vi "Secure-Release Region_01282025.vi"(6 "Numeric":dbl, 7 "Action":enum16{"Secure", "Release"}(ring), 8 "error in (no error)":errorcluster, 10 "Control In":T1={"I-O.lvclass"=refnum, "Gantry"=refnum, "Dispenser"="COM1"}, 11 "Carrier Tray in":refnum<class "Assembly Tray.lvclass">) -> (0 "error out":errorcluster, 1 "Position":i32, 2 "Control Out":T1={"I-O.lvclass"=refnum, "Gantry"=refnum, "Dispenser"="COM1"}, 3 "Carrier Tray out":refnum<class "Assembly Tray.lvclass">)   [LabVIEW 2021, in "Assembly Tray.lvclass"]
uses:
  Assembly Tray.lvclass
  C:/Users/User/Documents/Jessica_Code/Jessica_code_08062024/Gantry-CMU/UCSB-Gantry-HEP-main/Classes/Workspace/Fixture.lvclass
  Controller/Controllers.ctl
  Controller/I-O/I-O.lvclass
  C:/Program Files (x86)/Aerotech/A3200/LabVIEW/2010/Bin/Aerotech.A3200.dll
  Program Files (x86)/Aerotech/A3200/LabVIEW/2010/Bin/Aerotech.A3200.dll
  Fixture.lvclass/Fixture.ctl
  Assembly Tray.lvclass/Assembly Tray.ctl
  Fixture.lvclass
  Controller/Controller.lvclass
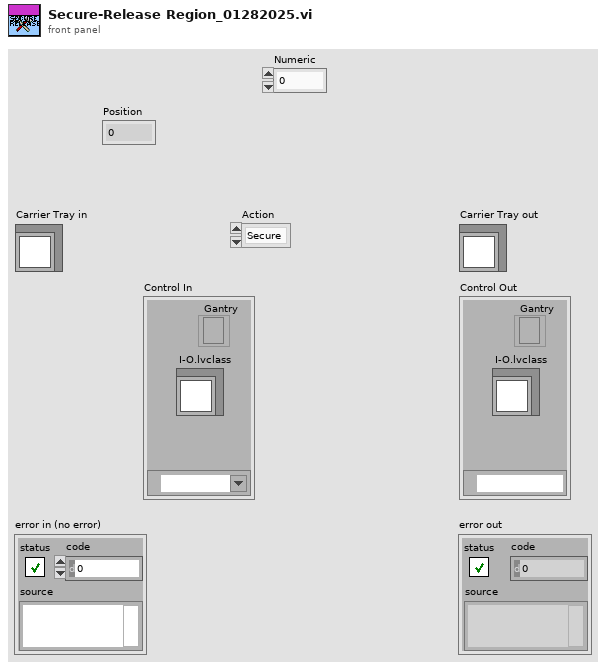
[diagram p1: front panel]
types:
  T1 = typedef "Controller.lvclass/Controllers.ctl" = cluster{"I-O.lvclass":refnum<class "I-O.lvclass">, "Gantry":refnum<k24>, "Dispenser":refnum<visa-resource-name>}
  T2 = typedef "I-O.lvclass/Pin Map.ctl" = cluster{"Region Valves":i32[], "Extra Valves":dbl[][][], "Tool Primary Valve":i32, "Tool Secondary Valve":i32, "Region Sensors":i32[], "Extra Sensors":dbl[][][], "Tool Primary Sensor":dbl, "Tool Secondary Sensor":dbl, "Compression Sensor":dbl, "5V":i32, "Dispenser Sensor":dbl}
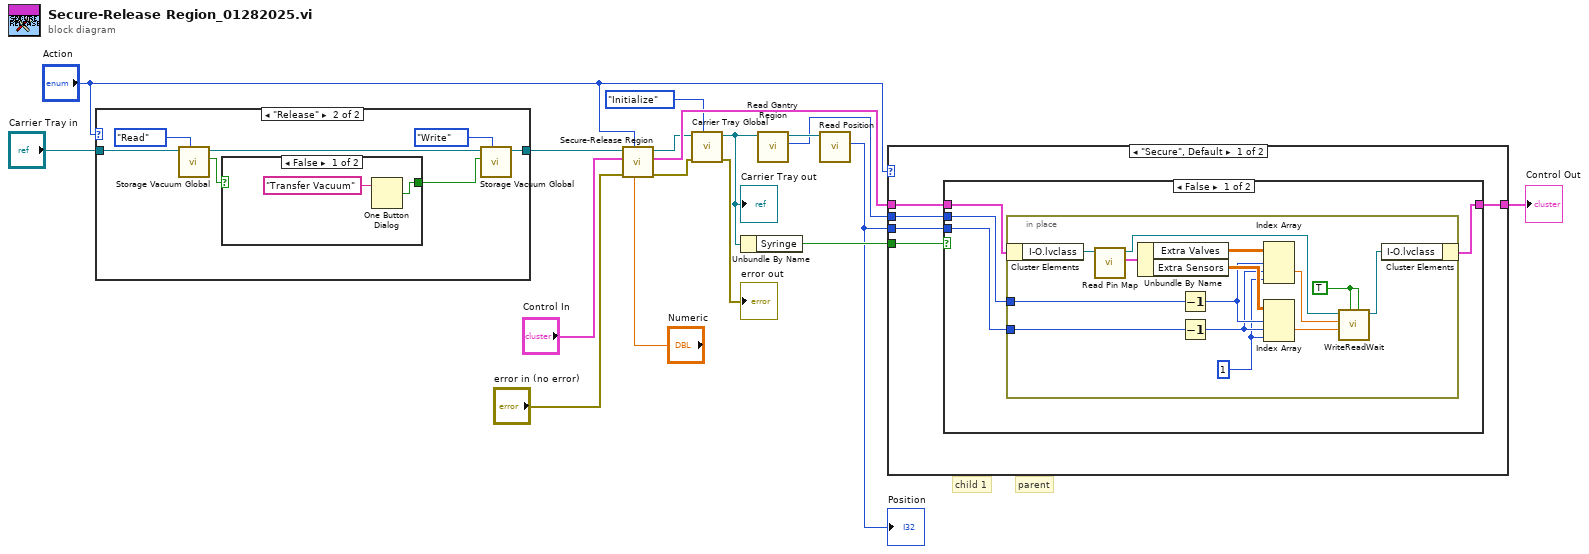
[diagram p0: block diagram]
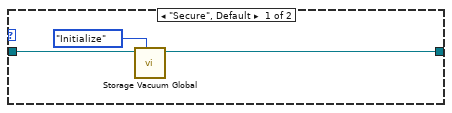
[diagram p4: hidden frame]
diagram:
  # "child 1"
  # "parent"
  n1 = case shown="\"Release\"" "Action" {
    tunnel: [w19 w22] -> w14
    tunnel: "Carrier Tray in" -> [w18 w21]
    frame "Secure", Default {
      n2 = call "Storage Vacuum Global.vi"("Action"=enum16{"Initialize", "Read", "Write"}."Initialize", "Carrier Tray.lvclass"=w18) -> ("Carrier Tray.lvclass 2"=w19:refnum<class "Assembly Tray.lvclass">)  [unwired: 7 in, 2 out]
    }
    frame "Release" {
      n3 = call "Storage Vacuum Global.vi"("Action"=enum16{"Initialize", "Read", "Write"}."Read", "Carrier Tray.lvclass"=w21) -> ("Read"=w27:bool, "Carrier Tray.lvclass 2"=w23:refnum<class "Assembly Tray.lvclass">)  [unwired: 7 in, 1 out]
      n4 = case shown="False" w27 {
        selector: w27 -> [_ w30]
        tunnel: [w28 w30] -> w24
        frame False {
          n5 = One Button Dialog(message="Transfer Vacuum") -> (true=w28:bool)  [unwired: 1 in]
        }
        frame True {
        }
      }
      n6 = call "Storage Vacuum Global.vi"("Action"=enum16{"Initialize", "Read", "Write"}."Write", "Write"=w24, "Carrier Tray.lvclass"=w23) -> ("Carrier Tray.lvclass 2"=w22:refnum<class "Assembly Tray.lvclass">)  [unwired: 6 in, 2 out]
    }
  }
  n7 = call-parent "Secure-Release Region.vi"("Test Run Number"="Numeric", "Action"="Action", "error in (no error)"="error in (no error)", "Control In"="Control In", "Fixture in"=w14) -> ("error out"=w4:errorcluster, "Control Out"=w12:T1, "Fixture out"=w7:refnum<class "Assembly Tray.lvclass">)  [unwired: 3 in, 1 out]
  n8 = call "Carrier Tray Global.vi"("Action"=enum16{"Initialize", "Read", "Write"}."Initialize", "error in (no error)"=w4, "Carrier Tray.lvclass"=w7) -> ("error out"=→"error out":errorcluster, "Carrier Tray.lvclass 2"=w6:refnum<class "Assembly Tray.lvclass">)  [unwired: 6 in, 1 out]
  "Carrier Tray out" <- w6
  n9 = Unbundle By Name(w6) -> ("Syringe"=w13:bool)
  n10 = call "Read Gantry Region.vi"("Fixture in"=w6) -> ("Gantry Region"=w10:i32, "Fixture out"=w11:refnum<class "Assembly Tray.lvclass">)  [unwired: 8 in, 1 out]
  n11 = call "Read Position.vi"("Fixture in"=w11) -> ("Position"=w2:i32)  [unwired: 8 in, 2 out]
  "Position" <- w2
  n12 = case shown="\"Secure\", Default" "Action" {
    tunnel: w13 -> [w35 _]
    tunnel: w12 -> [w34 w55]
    tunnel: w10 -> [w33 _]
    tunnel: w2 -> [w32 _]
    tunnel: [w31 w55] -> w9
    frame "Secure", Default {
      n13 = case shown="False" w35 {
        tunnel: w34 -> [w39 w54]
        tunnel: w33 -> [w38 _]
        tunnel: w32 -> [w37 _]
        tunnel: [w36 w54] -> w31
        frame False {
          n14 = in-place {
            in-place-border: w38 -> [w47]
            in-place-border: w37 -> [w45]
            w43 = 1
            w49 = TRUE
            n15 = in-place-cluster #1(w39) -> ("I-O.lvclass"=w53:refnum<class "I-O.lvclass">)
            n16 = call-dynamic "Read Pin Map.vi"("I-O in"=w53) -> ("Pin Map 2"=w52:T2, "I-O out"=w50:refnum<class "I-O.lvclass">)  [unwired: 8 in, 1 out]
            n17 = Unbundle By Name(w52) -> ("Extra Valves"=w40:dbl[][][], "Extra Sensors"=w51:dbl[][][])
            n18 = Decrement(x=w47) -> (x-1=w46:i32)
            n19 = Decrement(x=w45) -> (x-1=w44:i32)
            n20 = Index Array(array=w40, index (dim 0)=w46, index (dim 1)=w44, index (dim 2)=w43) -> (element=w42:dbl)
            n21 = Index Array(array=w51, index (dim 0)=w46, index (dim 1)=w44, index (dim 2)=w43) -> (element=w41:dbl)
            n22 = call "WriteReadWait.vi"("Read Value"=w49, "Write Value"=w49, "Read"=w41, "Write"=w42, "I-O in"=w50) -> ("I-O out"=w48:refnum<class "I-O.lvclass">)  [unwired: 5 in, 1 out]
            n23 = in-place-cluster #1("I-O.lvclass"=w48) -> (w36:T1)
          }
        }
        frame True {
        }
      }
    }
    frame "Release" {
    }
  }
  "Control Out" <- w9
